vi "AddSubMulDiv.vi"() -> ()   [LabVIEW 2015]
panel:
  in  "Stop Button":bool
  out "Answer":dbl
  in  "Y":dbl
  in  "X":dbl
  in  "Combo Box":string(combo)
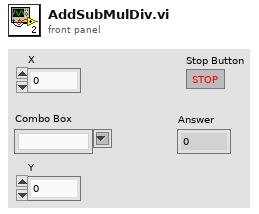
[diagram p1: front panel]
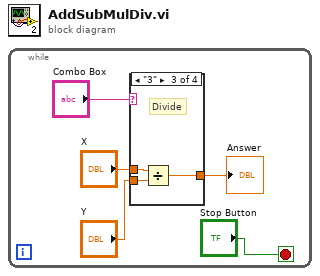
[diagram p0: block diagram]
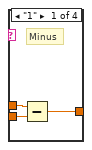
[diagram p2: hidden frame]
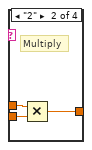
[diagram p3: hidden frame]
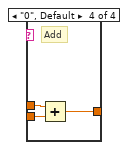
[diagram p4: hidden frame]
diagram:
  n1 = while {
    stop <- "Stop Button" stop-if-true
    n2 = case shown="\"3\"" "Combo Box" {
      tunnel: "X" -> [w8 w11 w14 w17]
      tunnel: "Y" -> [w7 w10 w13 w16]
      tunnel: [w6 w9 w12 w15] -> w2
      frame "1" {
        # "Minus"
        n3 = Subtract(x=w8, y=w7) -> (x-y=w6:dbl)
      }
      frame "2" {
        # "Multiply"
        n4 = Multiply(x=w11, y=w10) -> (x*y=w9:dbl)
      }
      frame "3" {
        # "Divide"
        n5 = Divide(x=w14, y=w13) -> (x/y=w12:dbl)
      }
      frame "0", Default {
        # "Add"
        n6 = Add(x=w17, y=w16) -> (x+y=w15:dbl)
      }
    }
    "Answer" <- w2
  }
